vi "Checks_Write Type Sequence.vi"(8 "error in (no error)":errorcluster, 11 "DMA":T1) -> (0 "error out":errorcluster)   [LabVIEW 2017, in "GE_RM_System Explorer.lvlib"]
doc: "This VI checks that, for a given DMA Write Block, all Relative Offset are present (no gap)."
uses:
  GE_RM_System Explorer.lvlib
  Typedef_DMA Instance.ctl
  Typedef_DMA Block Settings.ctl
  Shared/Data Channel Type.ctl
  Typedef_Channel Settings.ctl
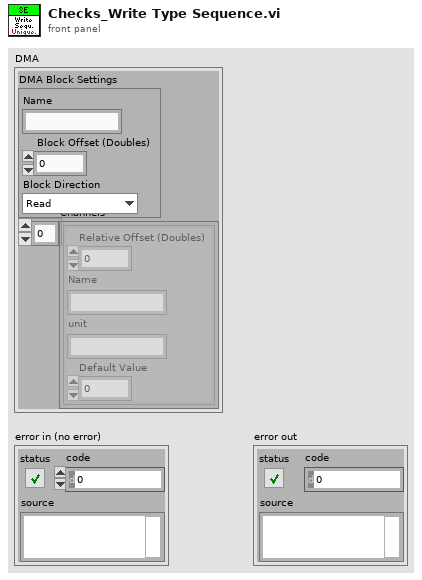
[diagram p1: front panel]
types:
  T1 = typedef "GE_RM_System Explorer.lvlib/Typedef_DMA Instance.ctl" = cluster{"DMA Block Settings":T2, "Channels":T4[]}
  T2 = typedef "GE_RM_System Explorer.lvlib/Typedef_DMA Block Settings.ctl" = cluster{"Name":string, " Block Offset (Doubles)":u32, "Block Direction":T3}
  T3 = typedef "GE_RM_System Explorer.lvlib/Data Channel Type.ctl" = enum16{"Read", "Write"}
  T4 = typedef "GE_RM_System Explorer.lvlib/Typedef_Channel Settings.ctl" = cluster{"Relative Offset (Doubles)":u32, "Name":string, "unit":string, "Default Value":dbl}
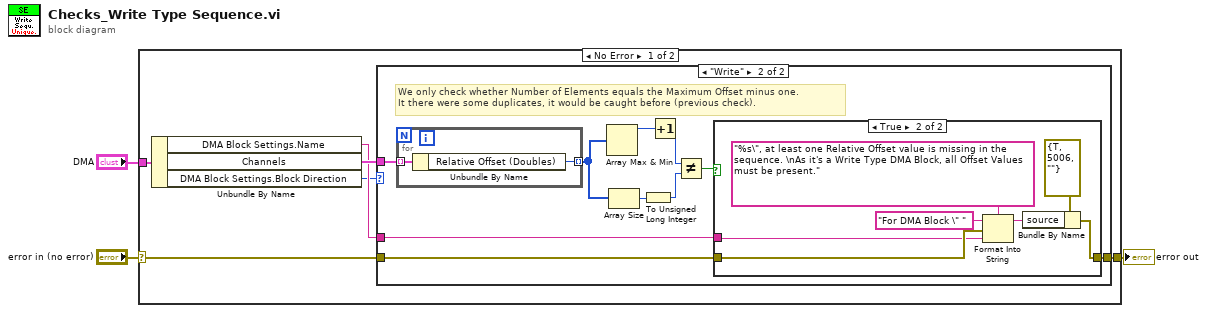
[diagram p0: block diagram]
diagram:
  n1 = case shown="No Error" "error in (no error)" {
    selector: "error in (no error)" -> [w7 w31]
    tunnel: [w6 w31] -> w3
    tunnel: "DMA" -> [w8 _]
    frame No Error {
      n2 = Unbundle By Name(w8) -> ("DMA Block Settings.Name"=w5:string, "Channels"=w9:T4[], "DMA Block Settings.Block Direction"=w4:T3)
      n3 = case shown="\"Write\"" w4 {
        tunnel: w9 -> [_ w20]
        tunnel: w7 -> [w10 w19]
        tunnel: [w10 w18] -> w6
        tunnel: w5 -> [_ w17]
        frame "Read", Default {
          # "We don't check that all elements are present for Read, it's not mandatory."
        }
        frame "Write" {
          # "We only check whether Number of Elements equals the Maximum Offset minus one.\nIt there were some duplicates, it would be caught before (previous check)."
          n4 = for {
            tunnel: w20 -> [w30] mode=indexing
            tunnel: [w29] -> w16 mode=indexing
            n5 = Unbundle By Name(w30) -> ("Relative Offset (Doubles)"=w29:u32)
          }
          n6 = Array Max & Min(array=w16) -> (max value=w15:u32)  [unwired: 3 out]
          n7 = Array Size(array=w16) -> (size(s)=w13:i32)
          n8 = To Unsigned Long Integer(number=w13) -> (unsigned 32bit integer=w11:u32)
          n9 = Increment(x=w15) -> (x+1=w12:u32)
          n10 = Not Equal?(x=w12, y=w11) -> (x != y?=w14:bool)
          n11 = case shown="True" w14 {
            tunnel: w19 -> [w21 w25]
            tunnel: [w21 w26] -> w18
            tunnel: w17 -> [_ w22]
            frame False {
            }
            frame True {
              n12 = Format Into String(format string="%s\", at least one Relative Offset value is missing in the sequence. \nAs it's a Write Type DMA Block, all Offset Values must be present.", initial string="For DMA Block \" ", error in=w25, w22) -> (resulting string=w27:string)  [unwired: 1 out]
              n13 = Bundle By Name(cluster=errorcluster {"status"=TRUE, "code"=5006, "source"=""} ("error IO"), "source"=w27) -> (w26:errorcluster)
            }
          }
        }
      }
    }
    frame Error {
    }
  }
  "error out" <- w3
